vi "Client References.vi"(7 "Comm ref":refnum<vi>, 10 "TestTimeout (0 ms)":i32, 11 "tcp listener ref":refnum<k5>) -> (3 "dup tcp listener ref":refnum<k5>)   [LabVIEW 2011]
uses:
  Client References.ctl
  Spartan Client Version.vi
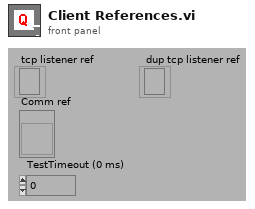
[diagram p1: front panel]
types:
  T1 = enum16{"Standard", "Buffered", "CRLF", "Immediate"}
  T2 = typedef "Client References.ctl" = cluster{"ID":string, "Test Reference":refnum<vi>, "In Use":bool, "Expire Time":timestamp}
  T3 = typedef "OGAB Version.ctl" = cluster{"Version":string, "Build Number":u32, "Build Date/Time":dbl}
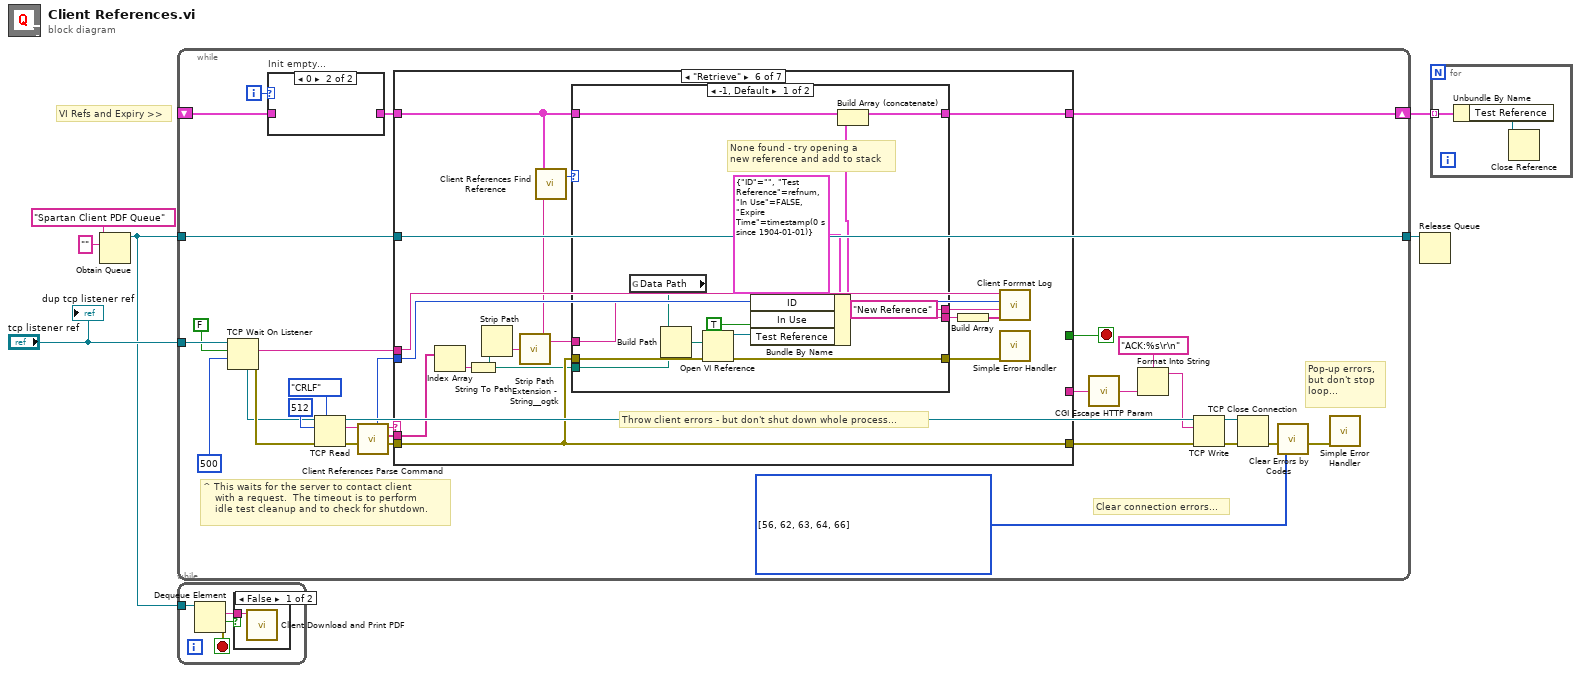
[diagram p0: block diagram]
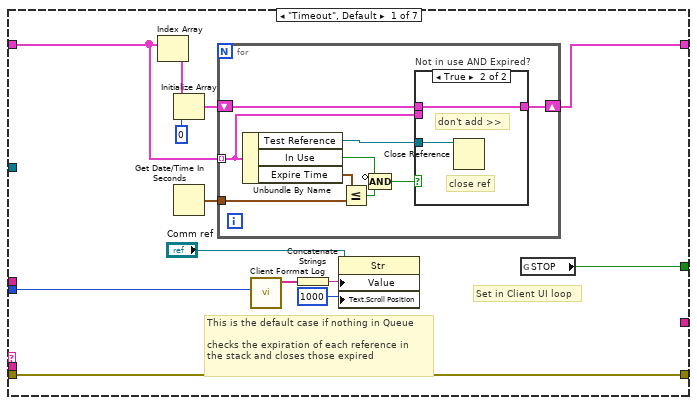
[diagram p4: hidden frame]
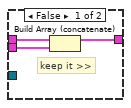
[diagram p5: hidden frame]
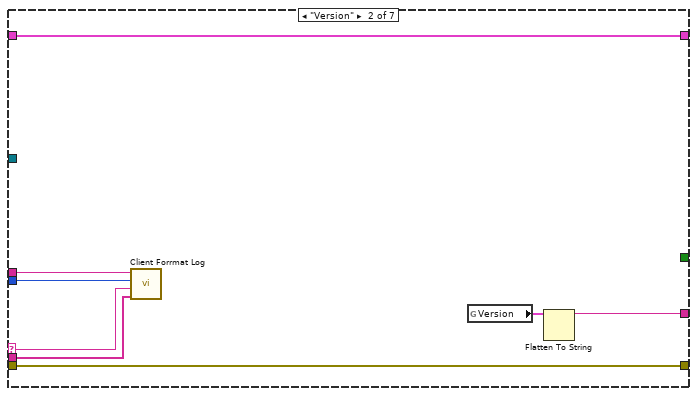
[diagram p6: hidden frame]
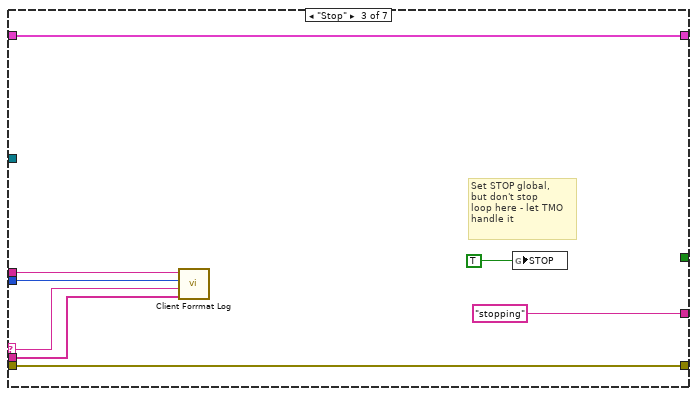
[diagram p7: hidden frame]
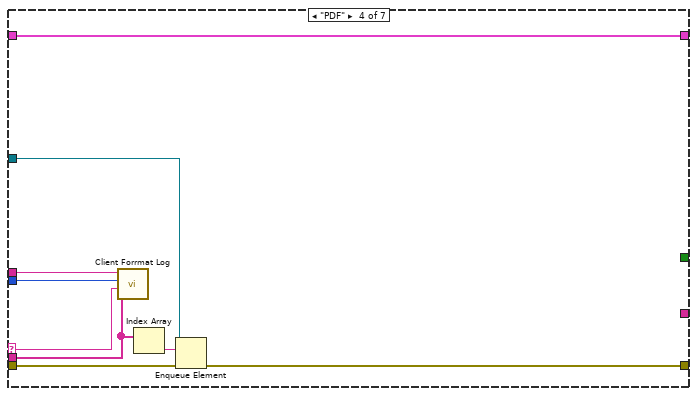
[diagram p8: hidden frame]
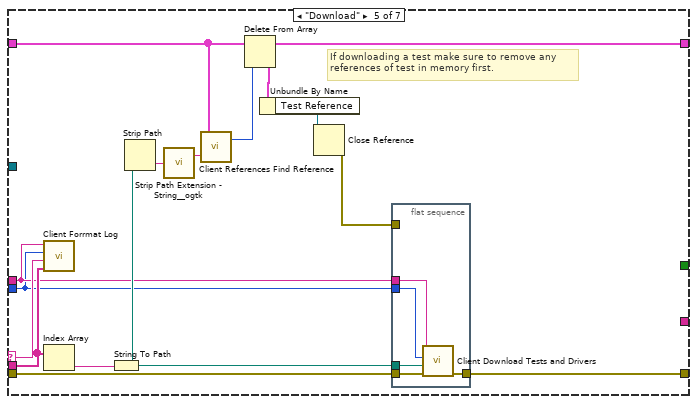
[diagram p9: hidden frame]
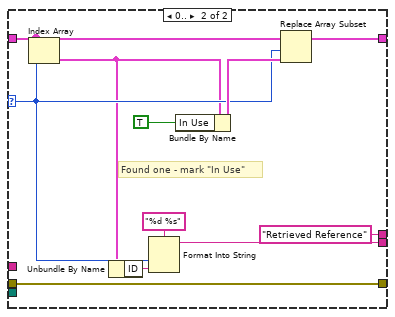
[diagram p10: hidden frame]
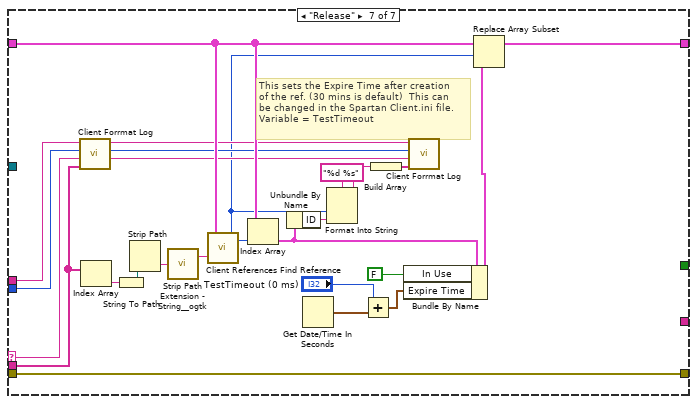
[diagram p11: hidden frame]
diagram:
  # "VI Refs and Expiry >>"
  n1 = Obtain Queue(name (unnamed)="Spartan Client PDF Queue", element data type="" ("name (unnamed)")) -> (queue out=w2:refnum<queue>)  [unwired: 3 in, 2 out]
  n2 = while {
    shift-right: [w36] -> w5
    shift-left: _ -> [w35]
    tunnel: "tcp listener ref" -> [w29]
    tunnel: w2 -> [w9]
    tunnel: [w9] -> w1
    i -> [w7]
    stop <- w13 stop-if-true
    w18 = i32[] [56, 62, 63, 64, 66] items=["No Error", "Argument Error", "Memory Full", "Out of Zone", "End of File", "File Already Open", "Generic File IO Error", "File Not Found", "File Permission Error", "Disk Full", "Duplicate Path", "Too Many Files Open", "Not Enabled", "Resource File Not Found", "Cannot Add Resource", "Resource Not Found", "Image Not Found", "Image Memory Error", "Pen Does Not Exist", "Config Bad Type", "Config Token Not Found", "Config Parse Error", "Config Memory Error", "Bad External Code Format", "Bad External Code Offset", "External Code Not Present", "Null Window", "Destroy Window Mixup", "Null Menu", "Print Aborted", "Bad Print Record", "Print Driver Error", "Windows Error During Print", "Memory Error During Print", "Print Dialog Error", "Generic Print Error", "Invalid Device Refnum", "Device Not Found", "Device Parameter Error", "Device Unit Error", "Can't Open Device", "Device Call Aborted", "Generic Error", "Cancelled By User", "Object ID Too Low", "Object ID Too High", "Object Not In Heap", "Unknown Heap", "Bad DefProc ID", "DefProc Not In Table", "Message Out Of Range", "Null Method", "Unknown Message", "Manager Call Not Supported", "Bad address", "Connection In progress", "Connection timed out", "Connection is already in progress", "Network attribute not supported", "Network error", "Address in use", "System out of memory", "Connection aborted", "Connection refused", "Connection is not connected", "Connection is already connected", "Connection closed", "Initialize error (interapplication manager)", "Bad occurrence", "Wait on unbound occurrence handler", "Occurrence queue overflow", "Bad path", "Semaphore not signaled", "Unrecognized type (interapplication manager)"]
    # "Pop-up errors,\nbut don't stop\nloop..."
    # "^ This waits for the server to contact client\n    with a request.  The timeout is to perform\n    idle test cleanup and to check for shutdown."
    # "Clear connection errors..."
    n3 = TCP Wait On Listener(9:500 ("timeout in ms (-1)"), 10:FALSE, 11:w29) -> (0:w28:errorcluster, 2:w10:string, 4:w25:refnum<k5>)  [unwired: 1 in, 2 out]
    n4 = case "Init empty..." shown="0" w7 {
      tunnel: w35 -> [w37 _]
      tunnel: [w37 _] -> w34
      frame Default {
      }
      frame 0 {
      }
    }
    n5 = TCP Read(connection ID=w25, bytes to read=512, error in (no error)=w28, 7:T1."CRLF" ("mode (standard)")) -> (connection ID out=w19:refnum<k5>, data out=w32:string, error out=w33:errorcluster)  [unwired: 1 out]
    n6 = call "Client References Parse Command.vi"("Queue Command (\"\")"=w32) -> ("Params"=w31:string[], "Function"=w11:string, "HTTP Port"=w8:u16)  [unwired: 8 out]
    n7 = case shown="\"Retrieve\"" w11 {
      selector: w11 -> [_ w68 w78 w88 w96 _ w155]
      tunnel: w33 -> [w46 w71 w79 w85 w105 w122 w171]
      tunnel: [w46 w71 w79 w84 w104 w122 w171] -> w21
      tunnel: [w49 w72 w80 w89 w102 w125 w167] -> w36
      tunnel: w34 -> [w45 w72 w80 w89 w103 w124 w166]
      tunnel: w31 -> [_ w67 w77 w87 w95 w113 w163]
      tunnel: w10 -> [_ w66 w74 w82 w93 w121 w158]
      tunnel: [_ w69 "stopping" _ _ _ _] -> w15
      tunnel: [w40 _ _ _ _ _ _] -> w13
      tunnel: w9 -> [_ _ _ w86 _ _ _]
      tunnel: w8 -> [w38 w65 w73 w81 w92 w120 w157]
      frame "Timeout", Default {
        # "Set in Client UI loop"
        # "This is the default case if nothing in Queue\n\nchecks the expiration of each reference in\nthe stack and closes those expired"
        n8 = Index Array(array=w45) -> (element=w44:T2)  [unwired: 1 in]
        n9 = Initialize Array(w44, 0 ("dimension size")) -> (w47:T2[])
        n10 = Get Date/Time In Seconds() -> (seconds since 1Jan1904=w50:timestamp)
        n11 = for {
          tunnel: w45 -> [w55] mode=indexing
          tunnel: w50 -> [w58]
          shift-right: [w56] -> w49
          shift-left: w47 -> [w57]
          n12 = Unbundle By Name(w55) -> ("Test Reference"=w51:refnum<vi>, "In Use"=w52:bool, "Expire Time"=w59:timestamp)
          n13 = Less Or Equal?(x=w59, y=w58) -> (x <= y?=w54:bool)
          n14 = Compound Arithmetic op=AND(invert w52, w54) -> (w53:bool)
          n15 = case "Not in use AND Expired?" shown="True" w53 {
            tunnel: w57 -> [w62 w64]
            tunnel: [w60 w64] -> w56
            tunnel: w55 -> [w61 _]
            tunnel: w51 -> [_ w63]
            frame False {
              # "keep it >>"
              n16 = Build Array (concatenate)(w62, w61) -> (w60:T2[])
            }
            frame True {
              # "close ref"
              # "don't add >>"
              n17 = Close Reference(reference=w63) -> ()  [unwired: 1 in, 1 out]
            }
          }
        }
        n18 = call "Client Forrmat Log.vi"("ServerPort (80)"=w38) -> ("Log"=w39:string[])  [unwired: 3 in, 7 out]
        n19 = Concatenate Strings(w39) -> (w43:string)
        n20 = property on="Property Node" class="Str"(reference="Comm ref", "Value"=w43, "Text.Scroll Position"=u32 1000) -> ()  [unwired: 1 in, 2 out]
        n21 = global read "Spartan Client Version.vi" "STOP"() -> (w40:bool)
      }
      frame "Version" {
        n22 = call "Client Forrmat Log.vi"("Params (empty)"=w67, "Command (\"\")"=w68, "ServerPort (80)"=w65, "SERVER (\"\")"=w66) -> ()  [unwired: 8 out]
        n23 = global read "Spartan Client Version.vi" "Version"() -> (w70:T3)
        n24 = Flatten To String(anything=w70) -> (data string=w69:string)  [unwired: 1 in, 4 out]
      }
      frame "Stop" {
        # "Set STOP global,\nbut don't stop\nloop here - let TMO\nhandle it"
        n25 = call "Client Forrmat Log.vi"("Params (empty)"=w77, "Command (\"\")"=w78, "ServerPort (80)"=w73, "SERVER (\"\")"=w74) -> ()  [unwired: 8 out]
        n26 = global write "Spartan Client Version.vi" "STOP"(TRUE) -> ()
      }
      frame "PDF" {
        n27 = call "Client Forrmat Log.vi"("Params (empty)"=w87, "Command (\"\")"=w88, "ServerPort (80)"=w81, "SERVER (\"\")"=w82) -> ()  [unwired: 8 out]
        n28 = Index Array(array=w87) -> (element=w83:string)  [unwired: 1 in]
        n29 = Enqueue Element(queue=w86, element=w83, error in (no error)=w85) -> (error out=w84:errorcluster)  [unwired: 3 out]
      }
      frame "Download" {
        # "If downloading a test make sure to remove any\nreferences of test in memory first."
        n30 = call "Client Forrmat Log.vi"("Params (empty)"=w95, "Command (\"\")"=w96, "ServerPort (80)"=w92, "SERVER (\"\")"=w93) -> ()  [unwired: 8 out]
        n31 = Index Array(array=w95) -> (element=w94:string)  [unwired: 1 in]
        n32 = String To Path(string=w94) -> (path=w97:path)
        n33 = Strip Path(path=w97) -> (name=w91:string)  [unwired: 1 out]
        n34 = call "Strip Path Extension - String__ogtk.vi"("path"=w91) -> ("root"=w90:string)  [unwired: 1 out]
        n35 = call "Client References Find Reference.vi"("ID to Find (\"\")"=w90, "TESTREFS (empty)"=w103) -> ("Element"=w101:i32)  [unwired: 1 out]
        n36 = Delete From Array(array=w103, index=w101) -> (deleted portion=w100:T2, array with subset deleted=w102:T2[])  [unwired: 1 in]
        n37 = Unbundle By Name(w100) -> ("Test Reference"=w99:refnum<vi>)
        n38 = Close Reference(reference=w99) -> (error out=w98:errorcluster)  [unwired: 1 in]
        n39 = flat-sequence {
          tunnel: w93 -> [w110]
          tunnel: w105 -> [w109]
          tunnel: [w108] -> w104
          tunnel: w97 -> [w107]
          tunnel: w98 -> [_]
          tunnel: w92 -> [w106]
          frame #0 {
            n40 = call "Client Download Tests and Drivers.vi"("error in (no error)"=w109, "Test or Driver URL Path (empty)"=w107, "ServerPort (80)"=w106, "Server (\"\")"=w110) -> ("error out"=w108:errorcluster)  [unwired: 7 out]
          }
        }
      }
      frame "Retrieve" {
        # "Throw client errors - but don't shut down whole process..."
        n41 = Index Array(array=w113) -> (element=w117:string)  [unwired: 1 in]
        n42 = String To Path(string=w117) -> (path=w116:path)
        n43 = Strip Path(path=w116) -> (name=w115:string)  [unwired: 1 out]
        n44 = call "Strip Path Extension - String__ogtk.vi"("path"=w115) -> ("root"=w114:string)  [unwired: 1 out]
        n45 = call "Client References Find Reference.vi"("ID to Find (\"\")"=w114, "TESTREFS (empty)"=w124) -> ("Element"=w119:i32)  [unwired: 1 out]
        n46 = case shown="-1, Default" w119 {
          selector: w119 -> [_ w141]
          tunnel: w122 -> [w138 w145]
          tunnel: [w137 w146] -> w125
          tunnel: w124 -> [w136 w147]
          tunnel: [w131 w145] -> w123
          tunnel: ["New Reference" "Retrieved Reference" ("message")] -> w118
          tunnel: w116 -> [w128 _]
          tunnel: w114 -> [w127 _]
          tunnel: [w127 w139] -> w112
          frame -1, Default {
            # "None found - try opening a \nnew reference and add to stack"
            n47 = global read "Spartan Client Version.vi" "Data Path"() -> (w126:path)
            n48 = Build Path(base path=w126, name or relative path=w128) -> (appended path=w130:path)
            n49 = Open VI Reference(vi path=w130, error in (no error)=w138) -> (vi reference=w132:refnum<vi>, error out=w131:errorcluster)  [unwired: 4 out]
            n50 = Bundle By Name(cluster=T2 {"ID"="", "Test Reference"=refnum, "In Use"=FALSE, "Expire Time"=timestamp(0 s since 1904-01-01)} ("Test Reference Cluster"), "ID"=w127, "In Use"=TRUE, "Test Reference"=w132) -> (w135:T2)
            n51 = Build Array (concatenate)(w136, w135) -> (w137:T2[])
          }
          frame 0.. {
            # "Found one - mark \"In Use\""
            n52 = Index Array(array=w147, index=w141) -> (element=w140:T2)
            n53 = Unbundle By Name(w140) -> ("ID"=w142:string)
            n54 = Format Into String(format string="%d %s", w141, w142) -> (resulting string=w139:string)  [unwired: 2 in, 1 out]
            n55 = Bundle By Name(cluster=w140, "In Use"=TRUE) -> (w149:T2)
            n56 = Replace Array Subset(array=w147, new element=w149, index=w141) -> (w146:T2[])
          }
        }
        n57 = Build Array(w112) -> (w111:string[])
        n58 = call "Client Forrmat Log.vi"("Params (empty)"=w111, "Command (\"\")"=w118, "ServerPort (80)"=w120, "SERVER (\"\")"=w121) -> ()  [unwired: 8 out]
        n59 = call <vilib>:"Simple Error Handler.vi"("error in (no error)"=w123) -> ()  [unwired: 1 in, 8 out]
      }
      frame "Release" {
        # "This sets the Expire Time after creation\nof the ref. (30 mins is default)  This can\nbe changed in the Spartan Client.ini file.\nVariable = TestTimeout"
        n60 = call "Client Forrmat Log.vi"("Params (empty)"=w163, "Command (\"\")"=w155, "ServerPort (80)"=w157, "SERVER (\"\")"=w158) -> ()  [unwired: 8 out]
        n61 = Index Array(array=w163) -> (element=w160:string)  [unwired: 1 in]
        n62 = String To Path(string=w160) -> (path=w162:path)
        n63 = Strip Path(path=w162) -> (name=w161:string)  [unwired: 1 out]
        n64 = call "Strip Path Extension - String__ogtk.vi"("path"=w161) -> ("root"=w159:string)  [unwired: 1 out]
        n65 = call "Client References Find Reference.vi"("ID to Find (\"\")"=w159, "TESTREFS (empty)"=w166) -> ("Element"=w152:i32)  [unwired: 1 out]
        n66 = Index Array(array=w166, index=w152) -> (element=w154:T2)
        n67 = Unbundle By Name(w154) -> ("ID"=w153:string)
        n68 = Get Date/Time In Seconds() -> (seconds since 1Jan1904=w165:timestamp)
        n69 = Format Into String(format string="%d %s", w152, w153) -> (resulting string=w151:string)  [unwired: 2 in, 1 out]
        n70 = Add(x="TestTimeout (0 ms)", y=w165) -> (x+y=w170:timestamp)
        n71 = Build Array(w151) -> (w150:string[])
        n72 = Bundle By Name(cluster=w154, "In Use"=FALSE, "Expire Time"=w170) -> (w168:T2)
        n73 = call "Client Forrmat Log.vi"("Params (empty)"=w150, "Command (\"\")"=w155, "ServerPort (80)"=w157, "SERVER (\"\")"=w158) -> ()  [unwired: 8 out]
        n74 = Replace Array Subset(array=w166, new element=w168, index=w152) -> (w167:T2[])
      }
    }
    n75 = call "CGI Escape HTTP Param.vi"("string"=w15) -> ("url-encoded string"=w14:string)
    n76 = Format Into String(format string="ACK:%s\r\n", w14) -> (resulting string=w17:string)  [unwired: 2 in, 1 out]
    n77 = TCP Write(connection ID=w19, data in=w17, error in (no error)=w21) -> (connection ID out=w20:refnum<k5>, error out=w22:errorcluster)  [unwired: 2 out]
    n78 = TCP Close Connection(connection ID=w20, error in (no error)=w22) -> (error out=w23:errorcluster)  [unwired: 2 out]
    n79 = call "Clear Errors by Codes.vi"("Error Codes\nto Clear (Empty)"=w18, "error in (no error)"=w23) -> ("error out"=w12:errorcluster)  [unwired: 5 out]
    n80 = call <vilib>:"Simple Error Handler.vi"("error in (no error)"=w12) -> ()  [unwired: 1 in, 8 out]
  }
  n81 = while {
    tunnel: w2 -> [w175]
    stop <- w174 stop-if-true
    n82 = Dequeue Element(queue=w175) -> (element=w172:string, timed out?=w173:bool, error out=w174:errorcluster)  [unwired: 1 in, 2 out]
    n83 = case shown="False" w173 {
      tunnel: w172 -> [w176 _]
      frame False {
        n84 = call "Client Download and Print PDF.vi"("PDF URL (\"\")"=w176) -> ()  [unwired: 1 in, 10 out]
      }
      frame True {
      }
    }
  }
  n85 = Release Queue(queue=w1) -> ()  [unwired: 1 in, 4 out]
  n86 = for {
    tunnel: w5 -> [w178] mode=indexing
    n87 = Unbundle By Name(w178) -> ("Test Reference"=w177:refnum<vi>)
    n88 = Close Reference(reference=w177) -> ()  [unwired: 1 in, 1 out]
  }
  "dup tcp listener ref" <- "tcp listener ref"
